vi "Describe Variant.vi"(11 "Variant":variant) -> (1 "Type Description":string, 2 "Description":string, 3 "Variant Description":string)   [LabVIEW 2020, in "Utilities.lvlib"]
uses:
  Utilities.lvlib
  <vilib>/Utility/Data Type/Type Definitions/Data Type.ctl
  <vilib>/Utility/Data Type/NI_Data Type.lvlib
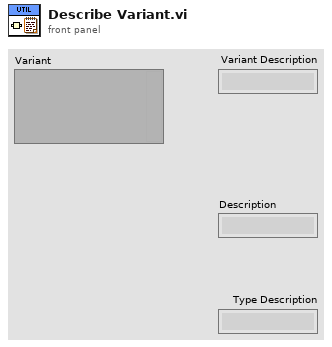
[diagram p1: front panel]
types:
  T1 = typedef "NI_Data Type.lvlib/Data Type.ctl" = enum8{"Invalid Type", "Void", "I8", "I16", "I32", "I64", "U8", "U16", "U32", "U64", "Single Float", "Double Float", "Extended Float", "Single Complex", "Double Complex", "Extended Complex", "Enum U8", "Enum U16", "Enum U32", "Enum U64", "Single Float With Unit", "Double Float With Unit", "Extended Float With Unit", "Single Complex with Unit", "Double Complex with Unit", "Extended Complex with Unit", "Boolean", "String", "Path", "Picture", "Tag", "Array", "Cluster", "Variant", "LV Variant", "Waveform", "Timestamp", "Digital Waveform", "Digital Data", "ExpressData", "Refnum", "External Data", "VI", "Poly VI", "LabVIEW Class Instance", "Fixed Point", "Set Collection", "Map Collection"}
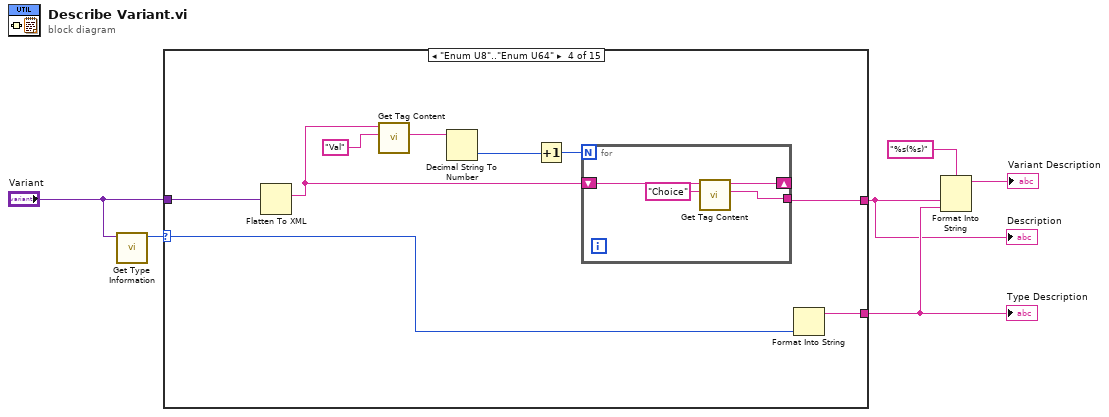
[diagram p0: block diagram]
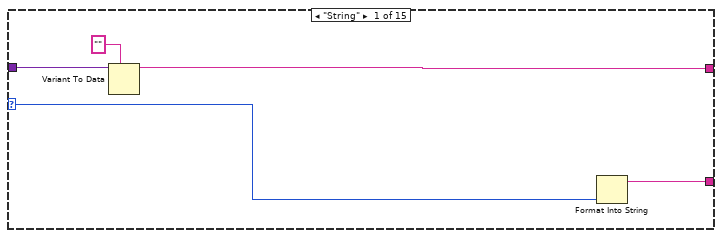
[diagram p2: hidden frame]
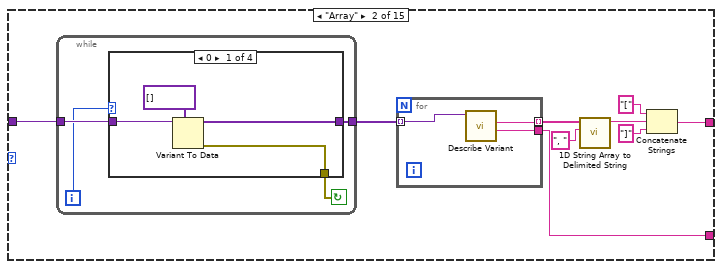
[diagram p3: hidden frame]
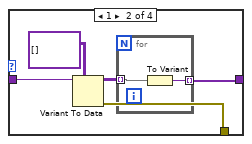
[diagram p4: hidden frame]
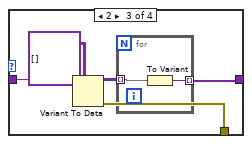
[diagram p5: hidden frame]
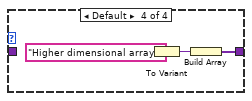
[diagram p6: hidden frame]
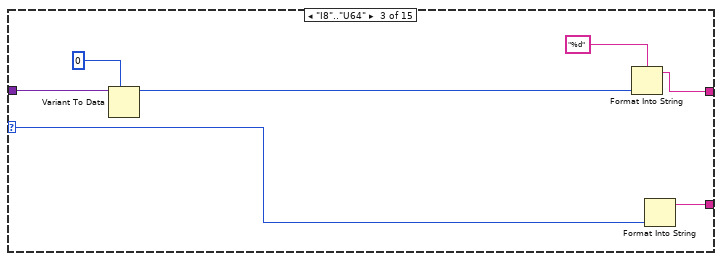
[diagram p7: hidden frame]
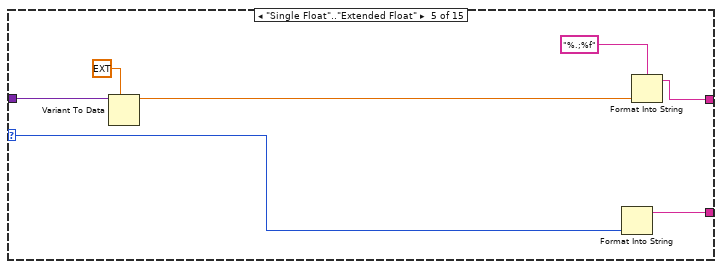
[diagram p8: hidden frame]
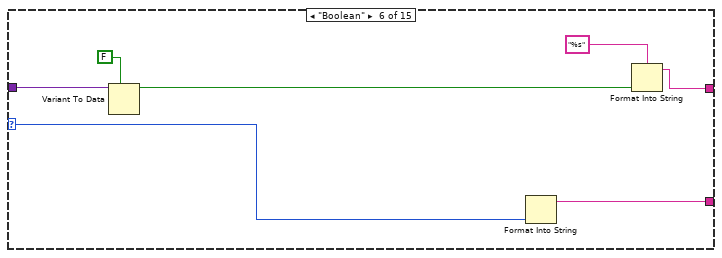
[diagram p9: hidden frame]
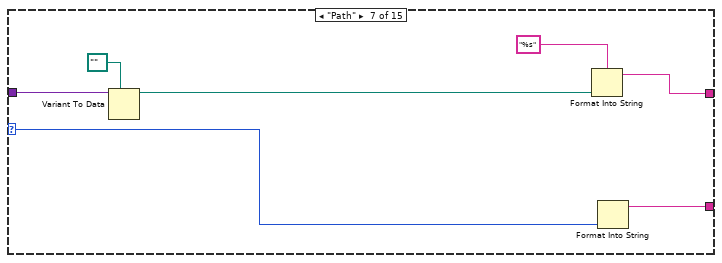
[diagram p10: hidden frame]
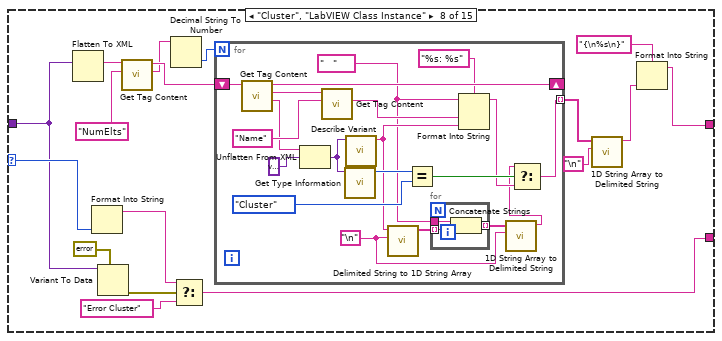
[diagram p11: hidden frame]
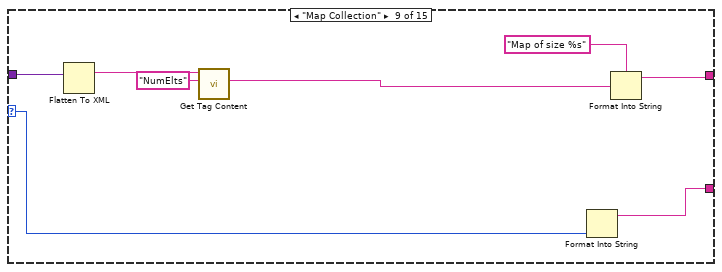
[diagram p12: hidden frame]
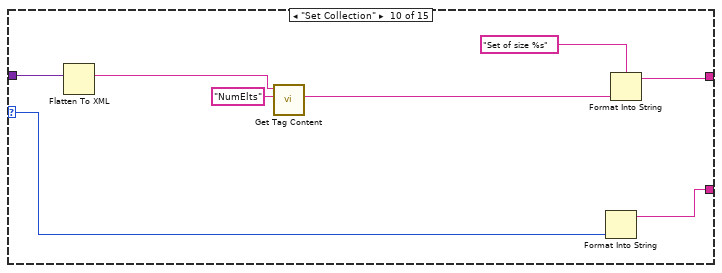
[diagram p13: hidden frame]
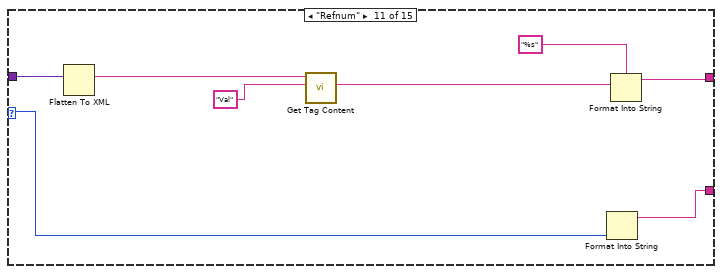
[diagram p14: hidden frame]
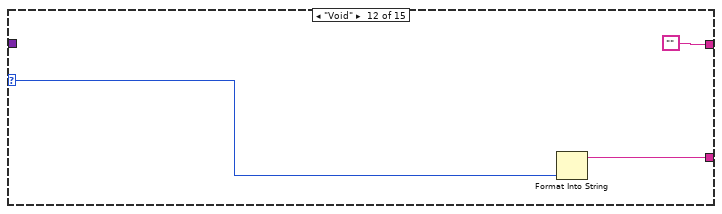
[diagram p15: hidden frame]
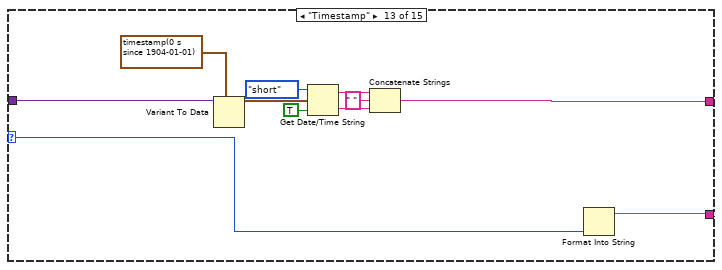
[diagram p16: hidden frame]
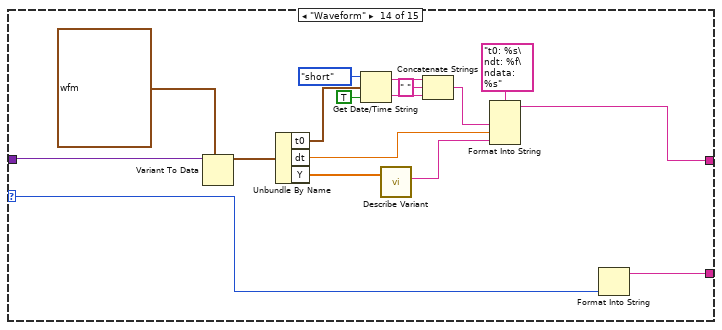
[diagram p17: hidden frame]
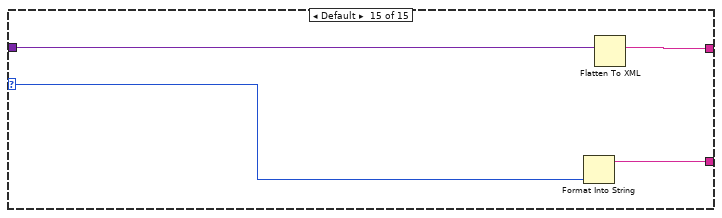
[diagram p18: hidden frame]
diagram:
  n1 = call <vilib>:"Get Type Information.vi"("variant"="Variant") -> ("type"=w5:T1)  [unwired: 6 in, 4 out]
  n2 = case shown="\"Enum U8\"..\"Enum U64\"" w5 {
    selector: w5 -> [w7 _ w49 w63 w69 w76 w83 w106 w133 w141 w149 w156 w167 w184 w185]
    tunnel: "Variant" -> [w11 w20 w55 w60 w75 w82 w89 w95 w137 w145 w153 _ w165 w182 w188]
    tunnel: [w10 w15 w51 w59 w71 w78 w85 w105 w135 w143 w151 "" w157 w168 w187] -> w2
    tunnel: [w8 w12 w50 w64 w70 w77 w84 w91 w134 w142 w150 w155 w166 w183 w186] -> w4
    frame "String" {
      n3 = Variant To Data(type="", Variant=w11) -> (data=w10:string)  [unwired: 1 in, 1 out]
      n4 = Format Into String(w7) -> (resulting string=w8:string)  [unwired: 3 in, 1 out]
    }
    frame "Array" {
      n5 = while {
        tunnel: w20 -> [w24]
        tunnel: [w23] -> w19
        i -> [w22]
        stop <- w21 continue-if-true
        n6 = case shown="0" w22 {
          tunnel: w24 -> [w28 w33 w40 _]
          tunnel: [w26 w30 w37 w43] -> w23
          tunnel: [w25 w29 w36 _] -> w21
          frame 0 {
            n7 = Variant To Data(type=variant[] [], Variant=w28) -> (data=w26:variant[], error out=w25:errorcluster)  [unwired: 1 in]
          }
          frame 1 {
            n8 = Variant To Data(type=variant[][] [], Variant=w33) -> (data=w31:variant[][], error out=w29:errorcluster)  [unwired: 1 in]
            n9 = for {
              tunnel: w31 -> [w35] mode=indexing
              tunnel: [w34] -> w30 mode=indexing
              n10 = To Variant(anything=w35) -> (Variant=w34:variant)
            }
          }
          frame 2 {
            n11 = Variant To Data(type=variant[][][] [], Variant=w40) -> (data=w38:variant[][][], error out=w36:errorcluster)  [unwired: 1 in]
            n12 = for {
              tunnel: w38 -> [w42] mode=indexing
              tunnel: [w41] -> w37 mode=indexing
              n13 = To Variant(anything=w42) -> (Variant=w41:variant)
            }
          }
          frame Default {
            n14 = To Variant(anything="Higher dimensional array") -> (Variant=w44:variant)
            n15 = Build Array(w44) -> (w43:variant[])
          }
        }
      }
      n16 = for {
        tunnel: w19 -> [w48] mode=indexing
        tunnel: [w46] -> w17 mode=indexing
        tunnel: [w47] -> w12
        n17 = call "Describe Variant.vi"("Variant"=w48) -> ("Type Description"=w47:string, "Description"=w46:string)  [unwired: 8 in, 1 out]
      }
      n18 = call <vilib>:"1D String Array to Delimited String.vi"("delimiter"=", ", "string array"=w17) -> ("delimited string"=w16:string)  [unwired: 9 in]
      n19 = Concatenate Strings("[", w16, "]") -> (w15:string)
    }
    frame "I8".."U64" {
      n20 = Variant To Data(type=i64 0, Variant=w55) -> (data=w53:i64)  [unwired: 1 in, 1 out]
      n21 = Format Into String(format string="%d", w53) -> (resulting string=w51:string)  [unwired: 2 in, 1 out]
      n22 = Format Into String(w49) -> (resulting string=w50:string)  [unwired: 3 in, 1 out]
    }
    frame "Enum U8".."Enum U64" {
      n23 = Flatten To XML(6:w60) -> (2:w58:string)
      n24 = call "Get Tag Content.vi"("Tag"="Val" ("string"), "xml string in"=w58) -> ("Tag content"=w56:string)  [unwired: 7 in, 2 out]
      n25 = Decimal String To Number(string=w56) -> (number=w61:i32)  [unwired: 2 in, 1 out]
      n26 = Increment(x=w61) -> (x+1=w62:i32)
      n27 = for {
        N: w62 -> [_]
        shift-right: [w67] -> _
        shift-left: w58 -> [w68]
        tunnel: [w66] -> w59
        n28 = call "Get Tag Content.vi"("Tag"="Choice", "xml string in"=w68) -> ("Tag content"=w66:string, "After end of tag"=w67:string)  [unwired: 7 in, 1 out]
      }
      n29 = Format Into String(w63) -> (resulting string=w64:string)  [unwired: 3 in, 1 out]
    }
    frame "Single Float".."Extended Float" {
      n30 = Variant To Data(type=ext 0.0, Variant=w75) -> (data=w73:ext)  [unwired: 1 in, 1 out]
      n31 = Format Into String(w69) -> (resulting string=w70:string)  [unwired: 3 in, 1 out]
      n32 = Format Into String(format string="%.;%f", w73) -> (resulting string=w71:string)  [unwired: 2 in, 1 out]
    }
    frame "Boolean" {
      n33 = Variant To Data(type=FALSE, Variant=w82) -> (data=w80:bool)  [unwired: 1 in, 1 out]
      n34 = Format Into String(w76) -> (resulting string=w77:string)  [unwired: 3 in, 1 out]
      n35 = Format Into String(format string="%s", w80) -> (resulting string=w78:string)  [unwired: 2 in, 1 out]
    }
    frame "Path" {
      n36 = Variant To Data(type=path "", Variant=w89) -> (data=w87:path)  [unwired: 1 in, 1 out]
      n37 = Format Into String(format string="%s", w87) -> (resulting string=w85:string)  [unwired: 2 in, 1 out]
      n38 = Format Into String(w83) -> (resulting string=w84:string)  [unwired: 3 in, 1 out]
    }
    frame "Cluster", "LabVIEW Class Instance" {
      n39 = Flatten To XML(6:w95) -> (2:w102:string)
      n40 = Format Into String(w106) -> (resulting string=w92:string)  [unwired: 3 in, 1 out]
      n41 = Variant To Data(type=errorcluster {"status"=FALSE, "code"=0, "source"=""} ("error constant"), Variant=w95) -> (error out=w93:errorcluster)  [unwired: 1 in, 1 out]
      n42 = call "Get Tag Content.vi"("Tag"="NumElts" ("regular expression"), "xml string in"=w102) -> ("Tag content"=w100:string, "After end of tag"=w101:string)  [unwired: 7 in, 1 out]
      n43 = Decimal String To Number(string=w100) -> (number=w99:i32)  [unwired: 2 in, 1 out]
      n44 = Select(t=w92, s=w93, f="Error Cluster") -> (s? t:f=w91:string)
      n45 = for {
        N: w99 -> [_]
        tunnel: [w113] -> w103 mode=indexing
        shift-right: [w125] -> _
        shift-left: w101 -> [w126]
        w108 = "\n"
        w110 = "   "
        n46 = call "Get Tag Content.vi"("xml string in"=w126) -> ("Tag with Content"=w119:string, "Tag content"=w122:string, "After end of tag"=w125:string)  [unwired: 8 in]
        n47 = Unflatten From XML(xml string=w119, type=variant) -> (value=w118:variant)  [unwired: 1 in, 1 out]
        n48 = call "Get Tag Content.vi"("Tag"="Name" ("regular expression"), "xml string in"=w122) -> ("Tag content"=w123:string)  [unwired: 7 in, 2 out]
        n49 = call <vilib>:"Get Type Information.vi"("variant"=w118) -> ("type"=w117:T1)  [unwired: 6 in, 4 out]
        n50 = call "Describe Variant.vi"("Variant"=w118) -> ("Variant Description"=w112:string)  [unwired: 8 in, 2 out]
        n51 = call <vilib>:"Delimited String to 1D String Array.vi"("delimiter"=w108, "delimited string"=w112) -> ("string array"=w111:string[])  [unwired: 9 in]
        n52 = Equal?(x=w117, y=Data_Type."Cluster" ("x")) -> (x = y?=w115:bool)
        n53 = for {
          tunnel: w111 -> [w129] mode=indexing
          tunnel: w110 -> [w128]
          tunnel: [w127] -> w109 mode=indexing
          n54 = Concatenate Strings(w128, w129) -> (w127:string)
        }
        n55 = Format Into String(format string="%s: %s", initial string=w110, w123, w112) -> (resulting string=w114:string)  [unwired: 1 in, 1 out]
        n56 = call <vilib>:"1D String Array to Delimited String.vi"("delimiter"=w108, "string array"=w109) -> ("delimited string"=w107:string)  [unwired: 9 in]
        n57 = Select(t=w107, s=w115, f=w114) -> (s? t:f=w113:string)
      }
      n58 = call <vilib>:"1D String Array to Delimited String.vi"("delimiter"="\n", "string array"=w103) -> ("delimited string"=w96:string)  [unwired: 9 in]
      n59 = Format Into String(format string="{\n%s\n}", w96) -> (resulting string=w105:string)  [unwired: 2 in, 1 out]
    }
    frame "Map Collection" {
      n60 = Flatten To XML(6:w137) -> (2:w131:string)
      n61 = call "Get Tag Content.vi"("Tag"="NumElts", "xml string in"=w131) -> ("Tag content"=w130:string)  [unwired: 7 in, 2 out]
      n62 = Format Into String(w133) -> (resulting string=w134:string)  [unwired: 3 in, 1 out]
      n63 = Format Into String(format string="Map of size %s", w130) -> (resulting string=w135:string)  [unwired: 2 in, 1 out]
    }
    frame "Set Collection" {
      n64 = Flatten To XML(6:w145) -> (2:w139:string)
      n65 = call "Get Tag Content.vi"("Tag"="NumElts", "xml string in"=w139) -> ("Tag content"=w138:string)  [unwired: 7 in, 2 out]
      n66 = Format Into String(w141) -> (resulting string=w142:string)  [unwired: 3 in, 1 out]
      n67 = Format Into String(format string="Set of size %s", w138) -> (resulting string=w143:string)  [unwired: 2 in, 1 out]
    }
    frame "Refnum" {
      n68 = Flatten To XML(6:w153) -> (2:w147:string)
      n69 = call "Get Tag Content.vi"("Tag"="Val" ("string"), "xml string in"=w147) -> ("Tag content"=w146:string)  [unwired: 7 in, 2 out]
      n70 = Format Into String(w149) -> (resulting string=w150:string)  [unwired: 3 in, 1 out]
      n71 = Format Into String(format string="%s", w146) -> (resulting string=w151:string)  [unwired: 2 in, 1 out]
    }
    frame "Void" {
      n72 = Format Into String(w156) -> (resulting string=w155:string)  [unwired: 3 in, 1 out]
    }
    frame "Timestamp" {
      n73 = Variant To Data(type=timestamp(0 s since 1904-01-01) ("current time"), Variant=w165) -> (data=w163:timestamp)  [unwired: 1 in, 1 out]
      n74 = Get Date/Time String(date format (0)=enum16{"short", "long", "abbreviated"}."short", seconds (now)=w163, want seconds? (F)=TRUE) -> (date string=w160:string, time string=w159:string)
      n75 = Concatenate Strings(w160, " " ("string"), w159) -> (w157:string)
      n76 = Format Into String(w167) -> (resulting string=w166:string)  [unwired: 3 in, 1 out]
    }
    frame "Waveform" {
      n77 = Variant To Data(type=waveform(dbl) {"t0"=timestamp(0 s since 1904-01-01), "dt"=1.0, "Y"=[]} ("Waveform"), Variant=w182) -> (data=w175:waveform(dbl))  [unwired: 1 in, 1 out]
      n78 = Unbundle By Name(w175) -> ("t0"=w174:timestamp, "dt"=w171:dbl, "Y"=w170:dbl[])
      n79 = Get Date/Time String(date format (0)=enum16{"short", "long", "abbreviated"}."short", seconds (now)=w174, want seconds? (F)=TRUE) -> (date string=w178:string, time string=w177:string)
      n80 = call "Describe Variant.vi"("Variant"=w170) -> ("Description"=w169:string)  [unwired: 8 in, 2 out]
      n81 = Concatenate Strings(w178, " " ("string"), w177) -> (w173:string)
      n82 = Format Into String(format string="t0: %s\ndt: %f\ndata: %s", w173, w171, w169) -> (resulting string=w168:string)  [unwired: 2 in, 1 out]
      n83 = Format Into String(w184) -> (resulting string=w183:string)  [unwired: 3 in, 1 out]
    }
    frame Default {
      n84 = Format Into String(w185) -> (resulting string=w186:string)  [unwired: 3 in, 1 out]
      n85 = Flatten To XML(6:w188) -> (2:w187:string)
    }
  }
  "Type Description" <- w4
  "Description" <- w2
  n86 = Format Into String(format string="%s(%s)", w2, w4) -> (resulting string=→"Variant Description":string)  [unwired: 2 in, 1 out]
